vi "Write Module path.vi"(8 "error in (no error)":errorcluster, 10 "Module path":path, 11 "Start-module in":refnum<class "Start-client.lvclass">) -> (0 "error out":errorcluster, 3 "Start-module out":refnum<class "Start-client.lvclass">)   [LabVIEW 2013, in "Messages.lvlib" / "Start-client.lvclass"]
uses:
  Start-client.lvclass
  Start-client.lvclass/Start-client.ctl
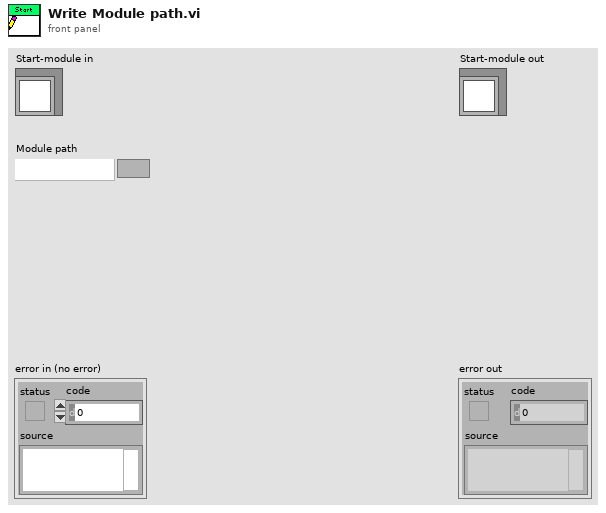
[diagram p1: front panel]
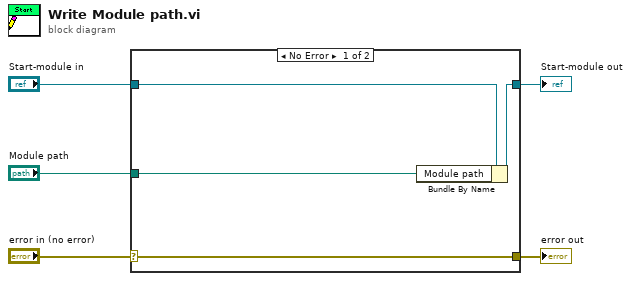
[diagram p0: block diagram]
diagram:
  n1 = case shown="No Error" "error in (no error)" {
    selector: "error in (no error)" -> [w9 w10]
    tunnel: [w9 w10] -> w4
    tunnel: [w7 w11] -> w2
    tunnel: "Start-module in" -> [w8 w11]
    tunnel: "Module path" -> [w6 _]
    frame No Error {
      n2 = Bundle By Name(cluster=w8, "Module path"=w6) -> (w7:refnum<class "Start-client.lvclass">)
    }
    frame Error {
    }
  }
  "error out" <- w4
  "Start-module out" <- w2
